vi "_RT_CtrlLoop_Manager.vi"(8 "error in (no error)":errorcluster, 10 "system state":refnum<data-value>, 11 "Signal Queue":refnum<queue>) -> ()   [LabVIEW 2018]
uses:
  PublicSubVI/Ctl/_ctl_RT_System_State.ctl
  PublicSubVI/Ctl/_ctl_RT_SysLog.ctl
  PublicSubVI/RS232/RS232ComPort.lvclass
  PublicSubVI/NewExpVar/ExpVar.lvclass
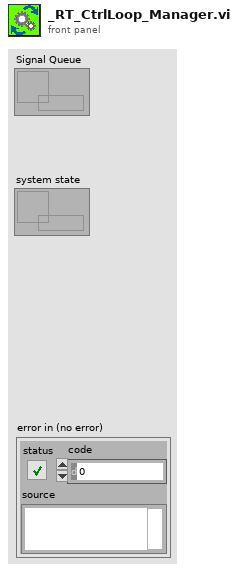
[diagram p1: front panel]
types:
  T1 = typedef "_ctl_RT_SysLog.ctl" = enum16{"None", "Initialize", "StartupRT", "StartupFPGA", "StartupAllocator", "GetMass", "SetWfmCode", "SetLaserCtrl", "SetTurboCtrl", "SetD999Ctrl", "Reconnecting...", "Interrupt", "StopRT"}
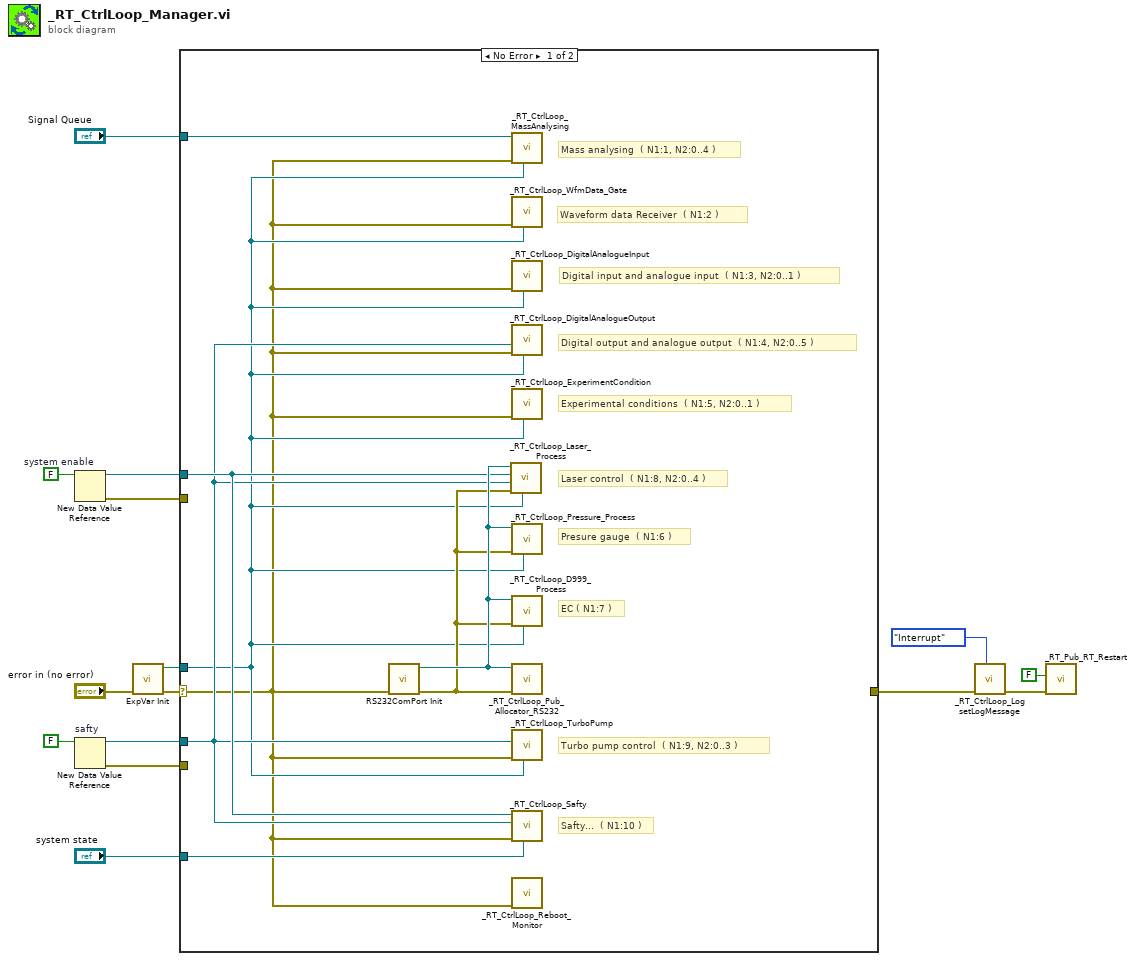
[diagram p0: block diagram]
diagram:
  n1 = New Data Value Reference "system enable"(data value=FALSE) -> (data value reference=w13:refnum<data-value>, error out=w12:errorcluster)  [unwired: 1 in]
  n2 = New Data Value Reference "safty"(data value=FALSE) -> (data value reference=w9:refnum<data-value>, error out=w8:errorcluster)  [unwired: 1 in]
  n3 = call "ExpVar Init.vi"("error in"="error in (no error)") -> ("error out"=w6:errorcluster, "NewExpVar.lvclass"=w5:refnum<class "ExpVar.lvclass">)  [unwired: 9 in]
  n4 = case shown="No Error" w6 {
    selector: w6 -> [w16 w24]
    tunnel: "Signal Queue" -> [w23 _]
    tunnel: [_ w24] -> w3
    tunnel: w13 -> [w19 _]
    tunnel: w12 -> [_ _]
    tunnel: "system state" -> [w20 _]
    tunnel: w9 -> [w18 _]
    tunnel: w8 -> [_ _]
    tunnel: w5 -> [w17 _]
    frame No Error {
      # "EC ( N1:7 )"
      # "Laser control  ( N1:8, N2:0..4 )"
      # "Presure gauge  ( N1:6 )"
      # "Waveform data Receiver  ( N1:2 )"
      # "Experimental conditions  ( N1:5, N2:0..1 )"
      # "Safty...  ( N1:10 )"
      # "Digital output and analogue output  ( N1:4, N2:0..5 )"
      # "Digital input and analogue input  ( N1:3, N2:0..1 )"
      # "Turbo pump control  ( N1:9, N2:0..3 )"
      # "Mass analysing  ( N1:1, N2:0..4 )"
      n5 = call "RS232ComPort Init.vi"("error in (no error)"=w16) -> ("error out"=w21:errorcluster, "RS232ComPort out"=w22:refnum<class "RS232ComPort.lvclass">)  [unwired: 9 in]
      n6 = call "_RT_CtrlLoop_Laser_Process.vi"("ExpVar in"=w17, "error in (no error)"=w21, "safty"=w18, "system enable"=w19, "RS232ComPort"=w22) -> ()  [unwired: 7 in]
      n7 = call "_RT_CtrlLoop_MassAnalysing.vi"("ExpVar in"=w17, "error in (no error)"=w16, "sig queue in"=w23) -> ()  [unwired: 9 in]
      n8 = call "_RT_CtrlLoop_WfmData_Gate.vi"("ExpVar in"=w17, "error in (no error)"=w16) -> ()  [unwired: 10 in]
      n9 = call "_RT_CtrlLoop_DigitalAnalogueInput.vi"("ExpVar in"=w17, "error in (no error)"=w16) -> ()  [unwired: 10 in]
      n10 = call "_RT_CtrlLoop_DigitalAnalogueOutput.vi"("ExpVar.lvclass"=w17, "error in (no error)"=w16, "safty"=w18) -> ()  [unwired: 9 in]
      n11 = call "_RT_CtrlLoop_ExperimentCondition.vi"("NewExpVar.lvclass"=w17, "error in"=w16) -> ()  [unwired: 9 in, 1 out]
      n12 = call "_RT_CtrlLoop_Pressure_Process.vi"("ExpVar.lvclass"=w17, "error in (no error)"=w21, "RS232ComPort In"=w22) -> ()  [unwired: 9 in]
      n13 = call "_RT_CtrlLoop_D999_Process.vi"("ExpVar in"=w17, "error in (no error)"=w21, "RS232ComPort in"=w22) -> ()  [unwired: 9 in]
      n14 = call "_RT_CtrlLoop_Pub_Allocator_RS232.vi"("error in (no error)"=w21, "RS232ComPort"=w22) -> ()  [unwired: 9 in, 1 out]
      n15 = call "_RT_CtrlLoop_TurboPump.vi"("ExpVar in"=w17, "error in (no error)"=w16, "safty"=w18) -> ()  [unwired: 9 in]
      n16 = call "_RT_CtrlLoop_Safty.vi"("system state"=w20, "error in (no error)"=w16, "safty"=w18, "system enable"=w19) -> ()  [unwired: 8 in]
      n17 = call "_RT_CtrlLoop_Reboot_Monitor.vi"("error in (no error)"=w16) -> ()  [unwired: 11 in]
    }
    frame Error {
    }
  }
  n18 = call "_RT_CtrlLoop_Log setLogMessage.vi"("system type"=_ctl_RT_SysLog."Interrupt", "error in"=w3) -> ("error out"=w2:errorcluster)  [unwired: 8 in, 1 out]
  n19 = call "_RT_Pub_RT_Restart.vi"("error in (no error)"=w2, "Safe Mode?"=FALSE) -> ()  [unwired: 9 in, 1 out]
